vi "instance count allowed.vi"(8 "error in":errorcluster, 11 "configuration in":refnum<class "action configuration.lvclass">) -> (0 "error out":errorcluster, 2 "instances allowed":i32, 3 "configuration out":refnum<class "action configuration.lvclass">)   [LabVIEW 2014, in "action configuration.lvclass"]
doc: "Provides an interface for determining the reentrancy of the runtime class associated with this configuration class. For example, a module which performs processing tasks may allow for unlimited instances (-1) while a component which implements a TCP server may want to limit itself to a smaller number in order to preserve ports. configuration.lvclass provides a value of 0, as no runtime class exists for this configuration."
uses:
  action configuration.lvclass
  <vilib>/NI/Tag Bus Module Framework/root configuration/TBM configuration.lvclass
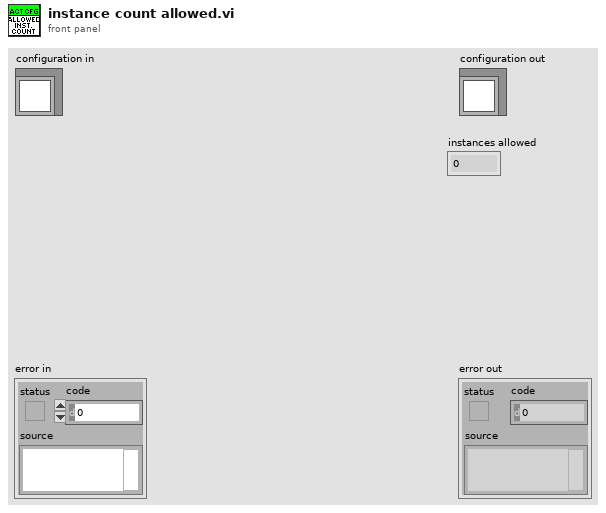
[diagram p1: front panel]
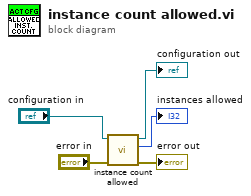
[diagram p0: block diagram]
diagram:
  n1 = call-parent "instance count allowed.vi"("error in"="error in", "configuration in"="configuration in") -> ("error out"=→"error out":errorcluster, "instances allowed"=→"instances allowed":i32, "configuration out"=→"configuration out":refnum<class "action configuration.lvclass">)  [unwired: 7 in]
